vi "_macro_Choreo_GetSwerveTrajectory.vi"() -> ()   [LabVIEW 2019, in "ChoreoLib.lvlib"]
uses:
  ChoreoLib.lvlib
  TypeDef/ChoreoTrajectorySwerve.ctl
  TypeDef/ChoreoSwerveSample.ctl
  TypeDef/ChoreoEventMarker.ctl
panel:
  out "ChoreoTrajectorySwerve":T1
  out "error out":errorcluster
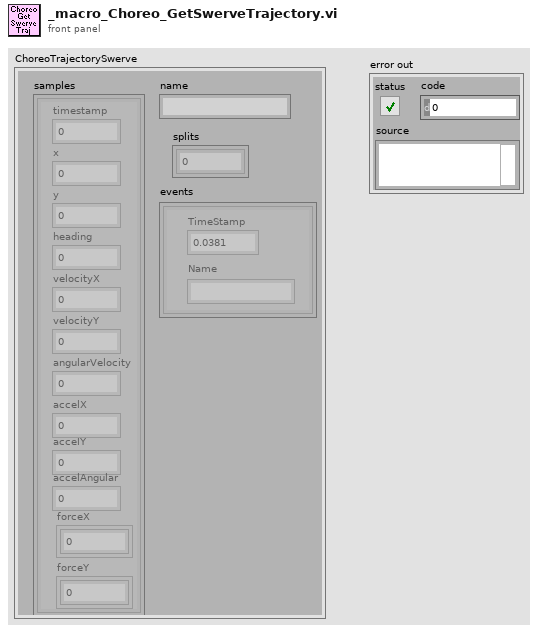
[diagram p1: front panel]
types:
  T1 = typedef "ChoreoLib.lvlib/ChoreoTrajectorySwerve.ctl" = cluster{"name":string, "samples":T2[], "splits":i32[], "events":T3[]}
  T2 = typedef "ChoreoLib.lvlib/ChoreoSwerveSample.ctl" = cluster{"timestamp":dbl, "x":dbl, "y":dbl, "heading":dbl, "velocityX":dbl, "velocityY":dbl, "angularVelocity":dbl, "accelX":dbl, "accelY":dbl, "accelAngular":dbl, "forceX":dbl[], "forceY":dbl[]}
  T3 = typedef "ChoreoLib.lvlib/ChoreoEventMarker.ctl" = cluster{"TimeStamp":dbl, "Name":string}
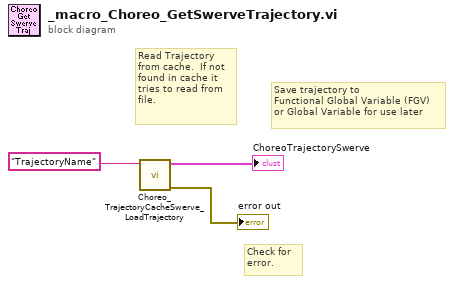
[diagram p0: block diagram]
diagram:
  # "Save trajectory to\nFunctional Global Variable (FGV)\nor Global Variable for use later"
  # "Check for \nerror."
  # "Read Trajectory\nfrom cache.  If not\nfound in cache it\ntries to read from\nfile."
  n1 = call "Choreo_TrajectoryCacheSwerve_LoadTrajectory.vi"("TrajectoryName"="TrajectoryName" ("FileName")) -> ("error out"=→"error out":errorcluster, "ChoreoTrajectorySwerve"=→"ChoreoTrajectorySwerve":T1)  [unwired: 9 in]
